vi "Read Piezo Voltage.vi"() -> ()   [LabVIEW 2012]
uses:
  <vilib>/DAQmx/create/channels.llb/DAQmx Create Channel (AI-Voltage-Basic).vi
  <vilib>/DAQmx/configure/timing.llb/DAQmx Timing (Sample Clock).vi
  <vilib>/DAQmx/read.llb/DAQmx Read (Analog Wfm 1Chan NSamp).vi
  <vilib>/DAQmx/create/channels.llb/DAQmx Create Channel (AO-Voltage-Basic).vi
  <vilib>/ptbypt/NI_PtbyPt.lvlib
  <vilib>/DAQmx/write.llb/DAQmx Write (Analog DBL 1Chan 1Samp).vi
panel:
  in  "Piezo Z":dbl=5.0 min=0.0 max=10.0 step=0.01
  out "z vs time":T1(graph)
  in  "Piezo Voltage":dbl=5.0 min=0.0 max=10.0 step=0.01
  in  "stop":bool
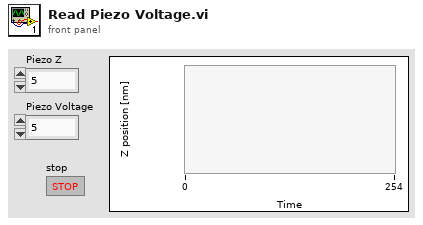
[diagram p1: front panel]
types:
  T1 = cluster{"Filtered x":dbl, "Z position":dbl, "Target Z [um]":dbl}
  T2 = cluster{"Filtered x":dbl, "data":waveform(dbl), "Piezo Voltage":dbl}
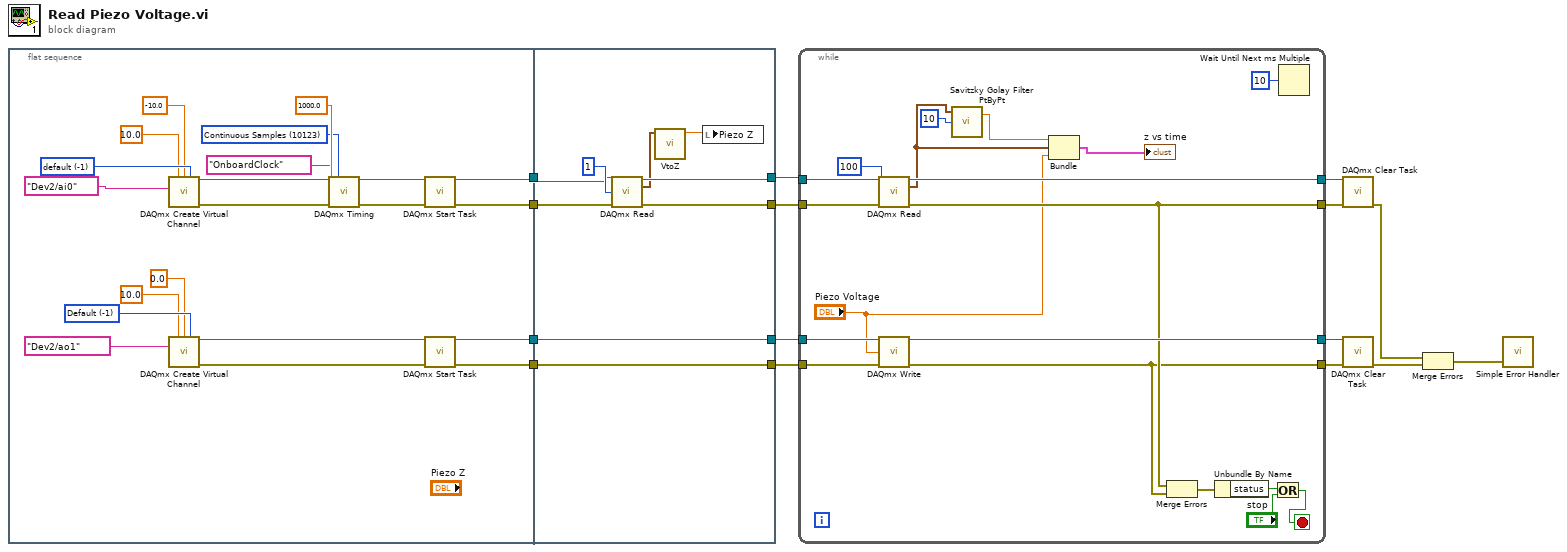
[diagram p0: block diagram]
diagram:
  n1 = flat-sequence {
    tunnel: [w25] -> w4
    tunnel: [w24] -> w3
    tunnel: [w17] -> w2
    tunnel: [w16] -> w1
    tunnel: [w40] -> w13
    tunnel: w4 -> [w42]
    tunnel: [w39] -> w12
    tunnel: w3 -> [w41]
    tunnel: [w45] -> w11
    tunnel: w2 -> [w45]
    tunnel: [w44] -> w10
    tunnel: w1 -> [w44]
    frame #0 {
      w22 = -1 items=["Default"=-1, "RSE"=10083, "Differential"=10106, "Pseudodifferential"=12529] ("output terminal configuration")
      w34 = 10123 items=["Finite Samples"=10178, "Continuous Samples"=10123, "Hardware Timed Single Point"=12522] ("sample mode")
      w28 = -1 items=["default"=-1, "RSE"=10083, "NRSE"=10078, "Differential"=10106, "Pseudodifferential"=12529] ("input terminal configuration")
      n2 = call-poly <vilib>:"DAQmx Create Virtual Channel.vi"("maximum value"=10.0, "minimum value"=-10.0, "input terminal configuration"=w28, "physical channels"=tag "Dev2/ai0" ("Physical Channel")) -> ("task out"=w30:refnum<k21>, "error out"=w29:errorcluster)  [unwired: 10 in]
      n3 = call-poly <vilib>:"DAQmx Create Virtual Channel.vi"("maximum value"=10.0, "minimum value"=0.0, "output terminal configuration"=w22, "physical channels"=tag "Dev2/ao1") -> ("task out"=w19:refnum<k21>, "error out"=w18:errorcluster)  [unwired: 10 in]
      n4 = call-poly <vilib>:"DAQmx Timing.vi"("task/channels in"=w30, "sample mode"=w34, "rate"=1000.0, "source"=tag "OnboardClock", "error in"=w29) -> ("task out"=w31:refnum<k21>, "error out"=w32:errorcluster)  [unwired: 9 in]
      n5 = call <vilib>:"DAQmx Start Task.vi"("task/channels in"=w31, "error in"=w32) -> ("task out"=w25:refnum<k21>, "error out"=w24:errorcluster)  [unwired: 12 in]
      n6 = call <vilib>:"DAQmx Start Task.vi"("task/channels in"=w19, "error in"=w18) -> ("task out"=w17:refnum<k21>, "error out"=w16:errorcluster)  [unwired: 12 in]
    }
    frame #1 {
      n7 = call-poly <vilib>:"DAQmx Read.vi"("task/channels in"=w42, "number of samples per channel"=1, "error in"=w41) -> ("task out"=w40:refnum<k21>, "data"=w38:waveform(dbl), "error out"=w39:errorcluster)  [unwired: 10 in]
      n8 = call "VtoZ.vi"("Voltage"=w38) -> ("Position"=w37:dbl)  [unwired: 10 in]
      n9 = local write "Piezo Z"(w37) -> ()
    }
  }
  n10 = while {
    tunnel: w13 -> [w64]
    tunnel: w12 -> [w63]
    tunnel: [w53] -> w15
    tunnel: [w62] -> w14
    tunnel: w11 -> [w60]
    tunnel: w10 -> [w59]
    tunnel: [w58] -> w9
    tunnel: [w52] -> w8
    stop <- w54 stop-if-true
    n11 = call-poly <vilib>:"DAQmx Read.vi"("task/channels in"=w64, "number of samples per channel"=100, "error in"=w63) -> ("task out"=w62:refnum<k21>, "data"=w49:waveform(dbl), "error out"=w53:errorcluster)  [unwired: 10 in]
    n12 = call-poly <vilib>:"DAQmx Write.vi"("task/channels in"=w60, "data"="Piezo Voltage", "error in"=w59) -> ("task out"=w58:refnum<k21>, "error out"=w52:errorcluster)  [unwired: 10 in, 1 out]
    n13 = call <vilib>:"Savitzky Golay Filter PtByPt.vi"("side points"=10, "x"=w49) -> ("Filtered x"=w47:dbl)  [unwired: 2 in, 1 out]
    n14 = Bundle("Filtered x"=w47, "data"=w49, "Piezo Voltage"="Piezo Voltage") -> (→"z vs time":T2)  [unwired: 1 in]
    n15 = Merge Errors(w53, w52) -> (w57:errorcluster)
    n16 = Unbundle By Name(w57) -> ("status"=w56:bool)
    n17 = Or(x=w56, y="stop") -> (x .or. y?=w54:bool)
    n18 = Wait Until Next ms Multiple(millisecond multiple=u32 10) -> ()  [unwired: 1 out]
  }
  n19 = call <vilib>:"DAQmx Clear Task.vi"("task in"=w14, "error in"=w15) -> ("error out"=w7:errorcluster)  [unwired: 13 in]
  n20 = call <vilib>:"DAQmx Clear Task.vi"("task in"=w9, "error in"=w8) -> ("error out"=w6:errorcluster)  [unwired: 13 in]
  n21 = Merge Errors(w7, w6) -> (w5:errorcluster)
  n22 = call <vilib>:"Simple Error Handler.vi"("error in (no error)"=w5) -> ()  [unwired: 4 in, 5 out]
